vi "OFDM_TransimitPreparation.vi"(10 "IQ rate":dbl, 11 "array":cdb[](array[numeric])) -> (3 "output cluster":cluster{"t0":dbl, "dt":dbl, "Y":cdb[]})   [LabVIEW 2014]
panel:
  out "size(s)":i32
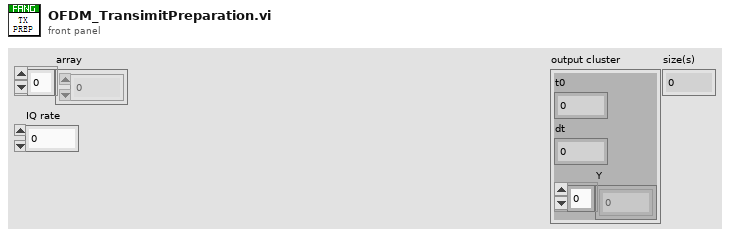
[diagram p1: front panel]
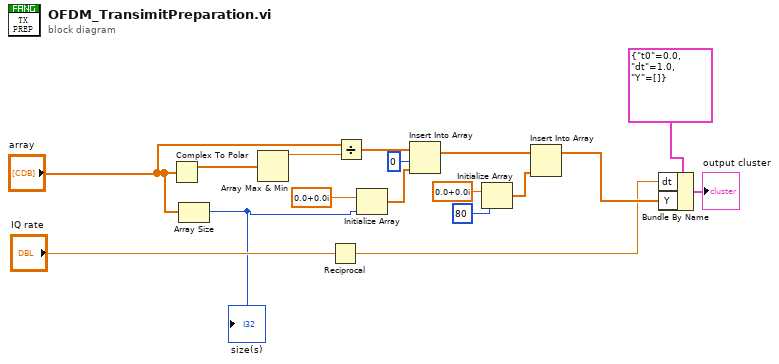
[diagram p0: block diagram]
diagram:
  n1 = Complex To Polar(r * e^(i*theta)="array") -> (r=w17:dbl[])  [unwired: 1 out]
  n2 = Array Size(array="array") -> (size(s)=w1:i32)
  "size(s)" <- w1
  n3 = Array Max & Min(array=w17) -> (max value=w16:dbl)  [unwired: 3 out]
  n4 = Reciprocal(x="IQ rate") -> (1/x=w3:dbl)
  n5 = Divide(x="array", y=w16) -> (x/y=w15:cdb[])
  n6 = Initialize Array(cdb 0.0+0.0i ("element"), w1) -> (w11:cdb[])
  n7 = Insert Into Array(array=w15, index=0, new element=w11) -> (w12:cdb[])
  n8 = Initialize Array(cdb 0.0+0.0i ("element"), 80 ("dimension size")) -> (w9:cdb[])
  n9 = Insert Into Array(array=w12, new element=w9) -> (w5:cdb[])  [unwired: 1 in]
  n10 = Bundle By Name(cluster=cluster{"t0":dbl, "dt":dbl, "Y":cdb[]} {"t0"=0.0, "dt"=1.0, "Y"=[]} ("data"), "dt"=w3, "Y"=w5) -> (→"output cluster":cluster{"t0":dbl, "dt":dbl, "Y":cdb[]})
